vi "Robot Global Data.vi"() -> ()   [LabVIEW 2013]
doc: "This global VI can contain as many global variables as you need. Place a control on the panel, give it a good name. To read or write to it from a VI, drag the icon to the diagram of that VI. You can also drag from the project. Click on the node to change which global you access. You shouldn't have multiple locations writing to a global or it will cause a race-condition."
uses:
  <vilib>/Rock Robotics/WPI/Camera/WPI_CameraImageSize.ctl
  <vilib>/Rock Robotics/WPI/DriverStation/WPI_DriverStationRobotMode2.ctl
panel:
  in  "Left Encoder":dbl=3.347870308
  in  "Right Encoder":dbl=3.347870308
  in  "inLow?":bool
  in  "WinchFireCount":i32=1
  in  "WinchPotPickUp":dbl=2.4
  in  "WinchDown":bool
  in  "Gear":T1={"RightLow"=137.0, "LeftLow"=147.0, "RightHigh"=83.0, "LeftHigh"=98.0}
  in  "HarvSetPoint":cluster{"Out":dbl, "In":dbl, "Clear":dbl}={"Out"=3.41, "In"=2.46, "Clear"=2.68}
  in  "WinchSetPointArray":T2={"Winch Desired Location"=2.19, "Winch Desired Location 2"=2.19, "Winch Desired Location 3"=2.19}
  in  "HarvClear":bool
  in  "HarvestStart":bool
  in  "WinchButPressed":bool
  in  "WinchCase":i32=2
  in  "Sorted Array":string[](array[string])
  in  "inAuton":bool
  in  "CamFireReady":bool
  out "CamPower":dbl
  in  "CamOutGearPos":dbl=3.5
  in  "CamInGearPos":dbl=4.1
  in  "CamPos":dbl=1.5
  in  "CamFire":bool
  out "HarvRoller":dbl
  out "HarvPower":dbl
  in  "HarvPot":dbl
  in  "WinchPower":dbl=1.0
  in  "Winch Pot Location":dbl=3.347870308
  out "Winch Motor Power Out":dbl
  out "Encoder":dbl
  out "Auton Array":dbl[][](array[numeric]) format="%0.3f"
  out "Current File":dbl
  out "Auton Files":string[](array[string])
  out "Number of Auton Files":dbl
  in  "Robot Mode":T3
  in  "LED toggle rate (ms)":u32=20
  in  "image size":T4=enum."320x240"
  in  "Enable Vision":bool
  # "Practice\nRL:137\nRH:83\nLL:147\nLH:98"
  # "Comp\nRL: 65\nRH: 110\nLL:110\nLH: 65"
  # "MAKE SURE TO\nCHECK THE COMP\nSETPOINTS IN\nDULUTH"
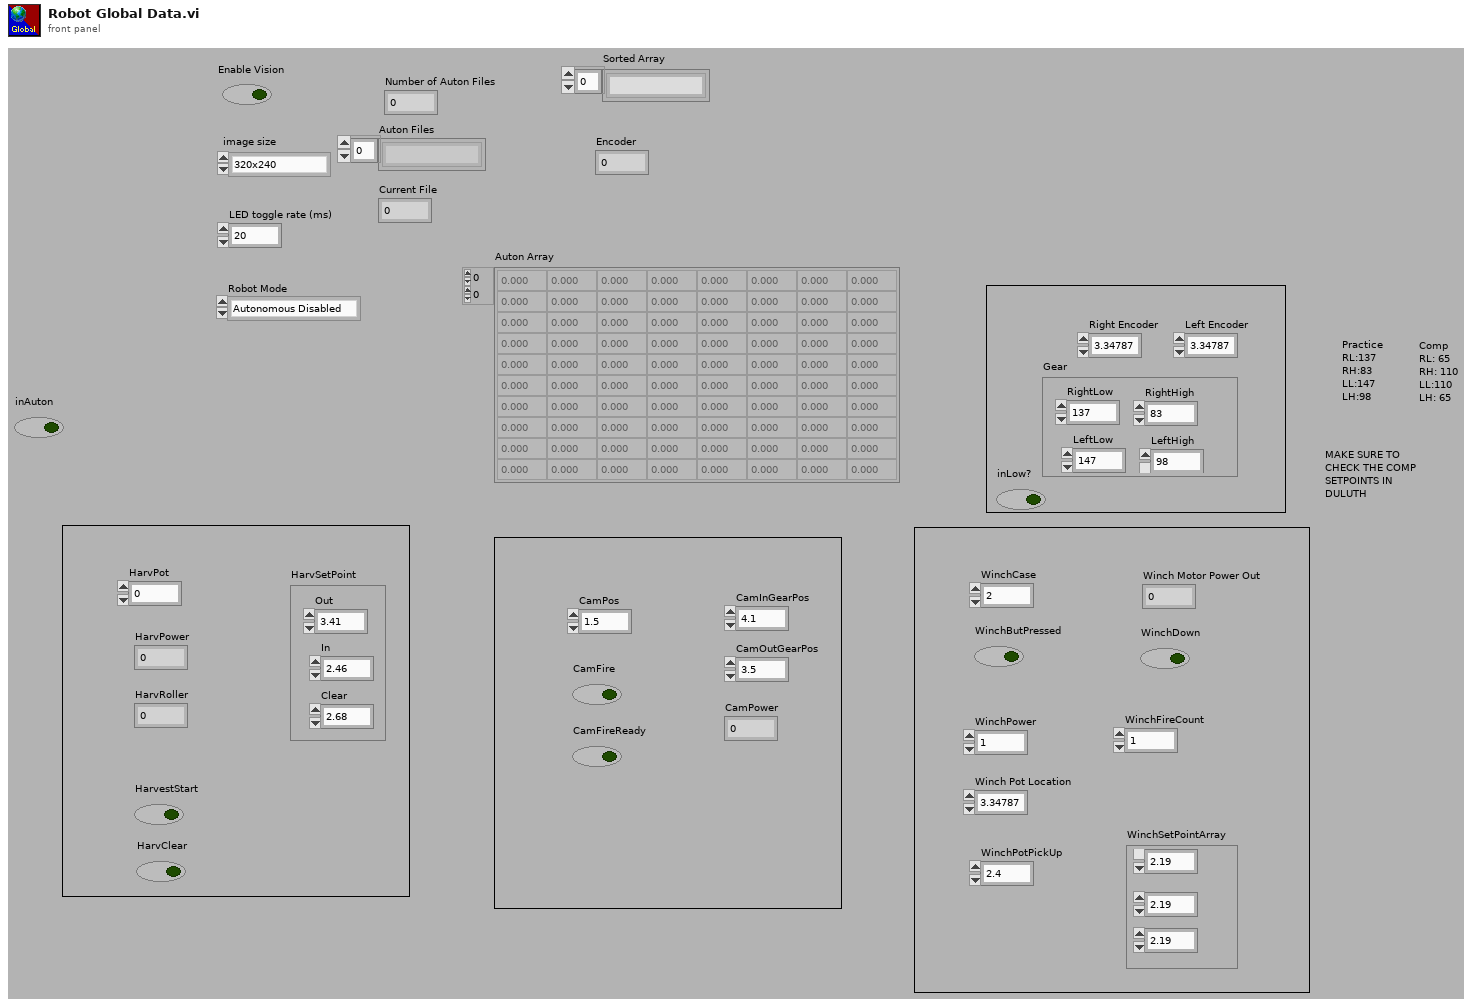
[diagram p1: front panel]
types:
  T1 = cluster{"RightLow":dbl, "LeftLow":dbl, "RightHigh":dbl, "LeftHigh":dbl}
  T2 = cluster{"Winch Desired Location":dbl, "Winch Desired Location 2":dbl, "Winch Desired Location 3":dbl}
  T3 = typedef "WPI_DriverStationRobotMode2.ctl" = enum16{"Autonomous Disabled", "Autonomous Enabled", "Teleop Disabled", "Teleop Enabled", "Timeout", "Finish", "Test Disabled", "Test Enabled"}
  T4 = typedef "WPI_CameraImageSize.ctl" = enum16{"640x480", "320x240", "160x120"}
diagram:
